vi "Process_EventLogger.vi"(8 "error in (no error)":errorcluster, 10 "MainApplication":refnum<class "MainApplication.lvclass">, 11 "Event Logger in":refnum<class "EventLogger.lvclass">) -> (0 "error out":errorcluster, 3 "Event Logger out":refnum<class "EventLogger.lvclass">)   [LabVIEW 2015, in "EventLogger.lvclass"]
uses:
  EventLogger.lvclass
  MainApplication/MainApplication.lvclass
  MainApplication/MainApplication.lvclass/MainApplication.ctl
  Controls/ChildToAppEventData.ctl
  MainApplication/Accessors/Read AppControlEvents.vi
  MainApplication/Accessors/Read MasterConfig.vi
  MainApplication/Accessors/Read QueueRefnums.vi
  MainApplication/Accessors/Read Dynamic CVT DVR.vi
  DAQ/DAQ.lvclass
  KDC/KDC.lvclass
  Shutter/Shutter.lvclass
  Laser/Laser.lvclass
  LinearStage/LinearStage.lvclass
  PowerMeter/PowerMeter.lvclass
  SystemUI/SystemUI.lvclass
  ChopperWheel/ChopperWheel.lvclass
  KST/KST.lvclass
panel:
  in  "StopLog":bool
  in  "StartLog":bool
  in  "OK":bool
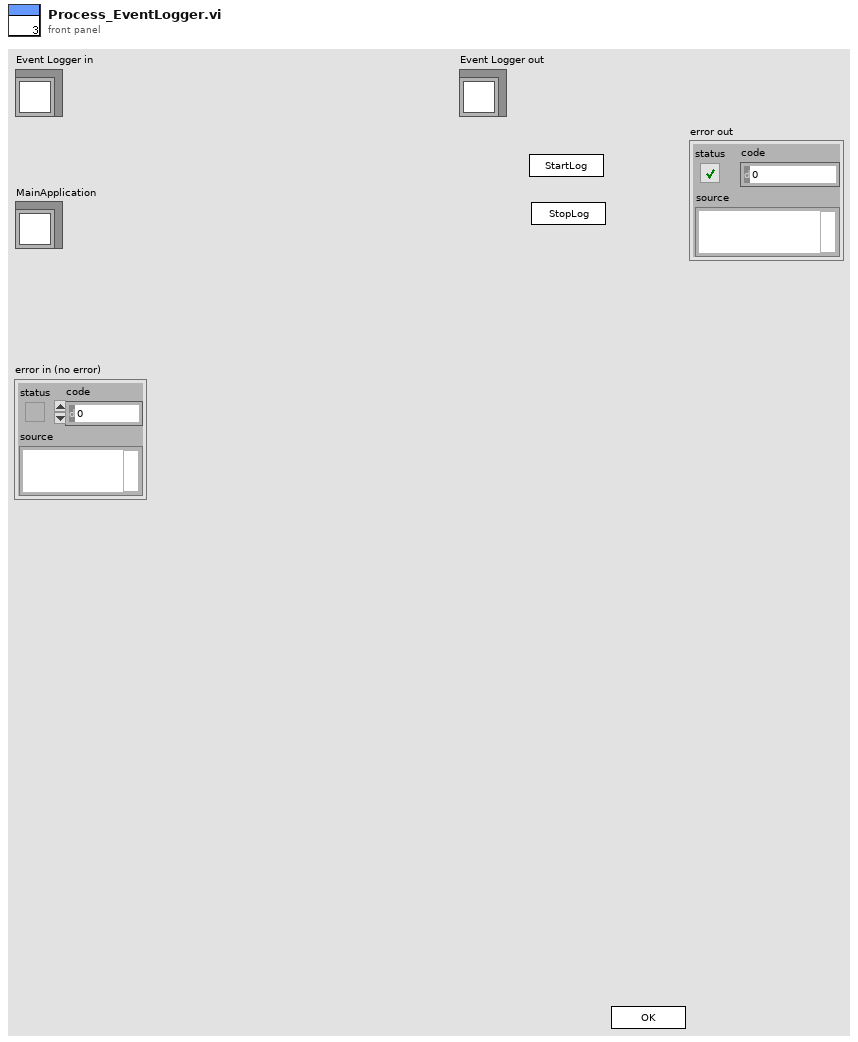
[diagram p1: front panel]
types:
  T1 = typedef "ChildToAppEventData.ctl" = cluster{"Command":string, "Data":variant}
  T2 = enum32{"invalid app kind", "Development System", "Run Time System", "Student Edition", "Embedded LabVIEW", "Evaluation", "Custom"}
  T3 = enum32{"Invalid", "Standard", "Closed", "Hidden", "Minimized", "Maximized"}
  T4 = typedef "PublicEvents--Cluster.ctl" = cluster{"AppToChildEvent":refnum<user-event>, "ChildToAppEvent":refnum<user-event>}
  T5 = typedef "MasterConfiguration--Cluster.ctl" = cluster{"MainAppConfiguration":T6, "ShutterConfiguration":T10, "KDCConfiguration":T12, "DAQConfiguration":T14, "LaserConfiguration":T18, "StageConfiguration":T20, "PowerMeterConfiguration":T22, "SystemUIConfiguration":T24, "ChopperWheelConfiguration":T26, "KSTConfiguration":T28, "Imaging":T30, "EventLoggerConfiguration":T31}
  T6 = typedef "MainAppConfiguration--Cluster.ctl" = cluster{"Simulate":bool, "Station Enable":T7, "StationNames":T8, "CustomScriptConfig":T9[], "C50":bool}
  T7 = typedef "StationEnable--Cluster.ctl" = cluster{"Station 1":bool, "Station 2":bool, "Station 3":bool, "Station 4":bool}
  T8 = typedef "StationModuleNames--Cluster.ctl" = cluster{"Station1Names":string[], "Station2Names":string[], "Station3Names":string[], "Station4Names":string[]}
  T9 = typedef "ScriptButtonConfig--cluster.ctl" = cluster{"OnScriptTitle":string, "OffScriptTitle":string, "OnScriptPath":path, "OffScriptPath":path}
  T10 = typedef "ShutterConfiguration--Cluster.ctl" = cluster{"Shutters":T11[]}
  T11 = typedef "SC10Config--Cluster.ctl" = cluster{"DeviceName":string, "Port":string, "Simulate":bool}
  T12 = typedef "KDC_Configuration--Cluster.ctl" = cluster{"KDC":T13[]}
  T13 = typedef "KDCConfig.ctl" = cluster{"SN":string, "S":dbl, "P":dbl, "Q":dbl, "DeviceName":string, "Simulation":bool, "Offset":dbl}
  T14 = typedef "DAQConfiguration--Cluster.ctl" = cluster{"DAQ":T15[], "Channels":T16[], "DOChannels":T17[]}
  T15 = typedef "DCON_Config--Cluster.ctl" = cluster{"Simulate":bool, "COM":refnum<visa-resource-name>, "baud":u32}
  T16 = typedef "ChannelProperties--Cluster.ctl" = cluster{"Name":string, "DeviceNo":string, "ChannelNo":string, "Active":bool}
  T17 = typedef "DO Channel Info--Cluster.ctl" = cluster{"Name":string, "DeviceNo":string, "GroupNo":string, "Active":bool}
  T18 = typedef "LaserConfiguration--Cluster.ctl" = cluster{"Laser":T19, "LaserLogFolderPath":path, "LaserLogNamePrefix":string, "LaserLogFileInterval_min":dbl, "LaserLogDataInterval_s":dbl}
  T19 = typedef "LaserConfig--Cluster.ctl" = cluster{"DeviceName":string, "Port":string, "Simulate":bool}
  T20 = typedef "LinearStageConfiguration--Cluster.ctl" = cluster{"Stage":T21}
  T21 = typedef "Stage_Config--Cluster.ctl" = cluster{"Simulate":bool, "COM":refnum<visa-resource-name>, "baud":u32}
  T22 = typedef "PowerMeterConfiguration--Cluster.ctl" = cluster{"PowerMeters":T23[], "DataFolderPath":path, "FileNamePrefix":string}
  T23 = typedef "PowerMeterDeviceConfig--Cluster.ctl" = cluster{"DeviceName":string, "SerialNumber":string, "Simulate":bool}
  T24 = typedef "SystemUIConfiguration--Cluster.ctl" = cluster{"Simulate":bool, "SystemUIParameters":T25}
  T25 = typedef "SystemUIParameters--Cluster.ctl" = cluster{"X center":dbl, "Y center":dbl, "X Size":dbl, "Y Size":dbl, "Gap Between Rows":dbl, "Gap Between Columns":dbl, "Gap Between Stage and Stations":dbl, "ConfigType":enum16{"Single-8", "Quad-8", "Quad-16"}}
  T26 = typedef "ChopperWheelConfiguration--Cluster.ctl" = cluster{"ChopperWheel":T27[]}
  T27 = typedef "MC2000B_DevConfig--Cluster.ctl" = cluster{"DeviceName":string, "COMPort":string, "Simulate":bool}
  T28 = typedef "KST_Configuration--Cluster.ctl" = cluster{"KST":T29[]}
  T29 = typedef "KSTConfig.ctl" = cluster{"SN":string, "S":dbl, "P":dbl, "Q":dbl, "DeviceName":string, "Simulation":bool, "Offset":dbl}
  T30 = typedef "Imaging--Cluster.ctl" = cluster{"Cam1":string, "Cam 2":string, "Cam 3":string}
  T31 = typedef "EventLogger_Configuration--Cluster.ctl" = cluster{"LogFolderPath":path}
  T32 = cluster{"Core":cluster{"Current VI Reference":refnum<vi>, "Close Panel on Exit?":bool}, "Event Logger in":refnum<class "EventLogger.lvclass">, "AppControlEvents":T4, "MasterConfiguration*":T5, "LaserConfiguration":T18, "Running":bool}
  T33 = cluster{"Current VI Reference":refnum<vi>, "Close Panel on Exit?":bool}
  T34 = typedef "MS Queue Cluster.ctl" = cluster{"MainQ":refnum<queue>, "StagesQ":refnum<queue>, "ShutterQ":refnum<queue>, "ZaberQ":refnum<queue>, "LaserD":refnum<queue>, "KDCQ":refnum<queue>, "Station 1":refnum<queue>, "Station 2":refnum<queue>, "Station 3":refnum<queue>, "Station 4":refnum<queue>, "PowerMeter":refnum<queue>, "DAQ":refnum<queue>, "CW":refnum<queue>, "KST":refnum<queue>, "EventLogger":refnum<queue>}
  T35 = typedef "TD Dynamic CVT DVR--ref.ctl" = refnum<data-value>
  T36 = cluster{"log file path":path, "Dynamic CVT":T35, "LogFolderPath":path, "Headers in Logfile":string[]}
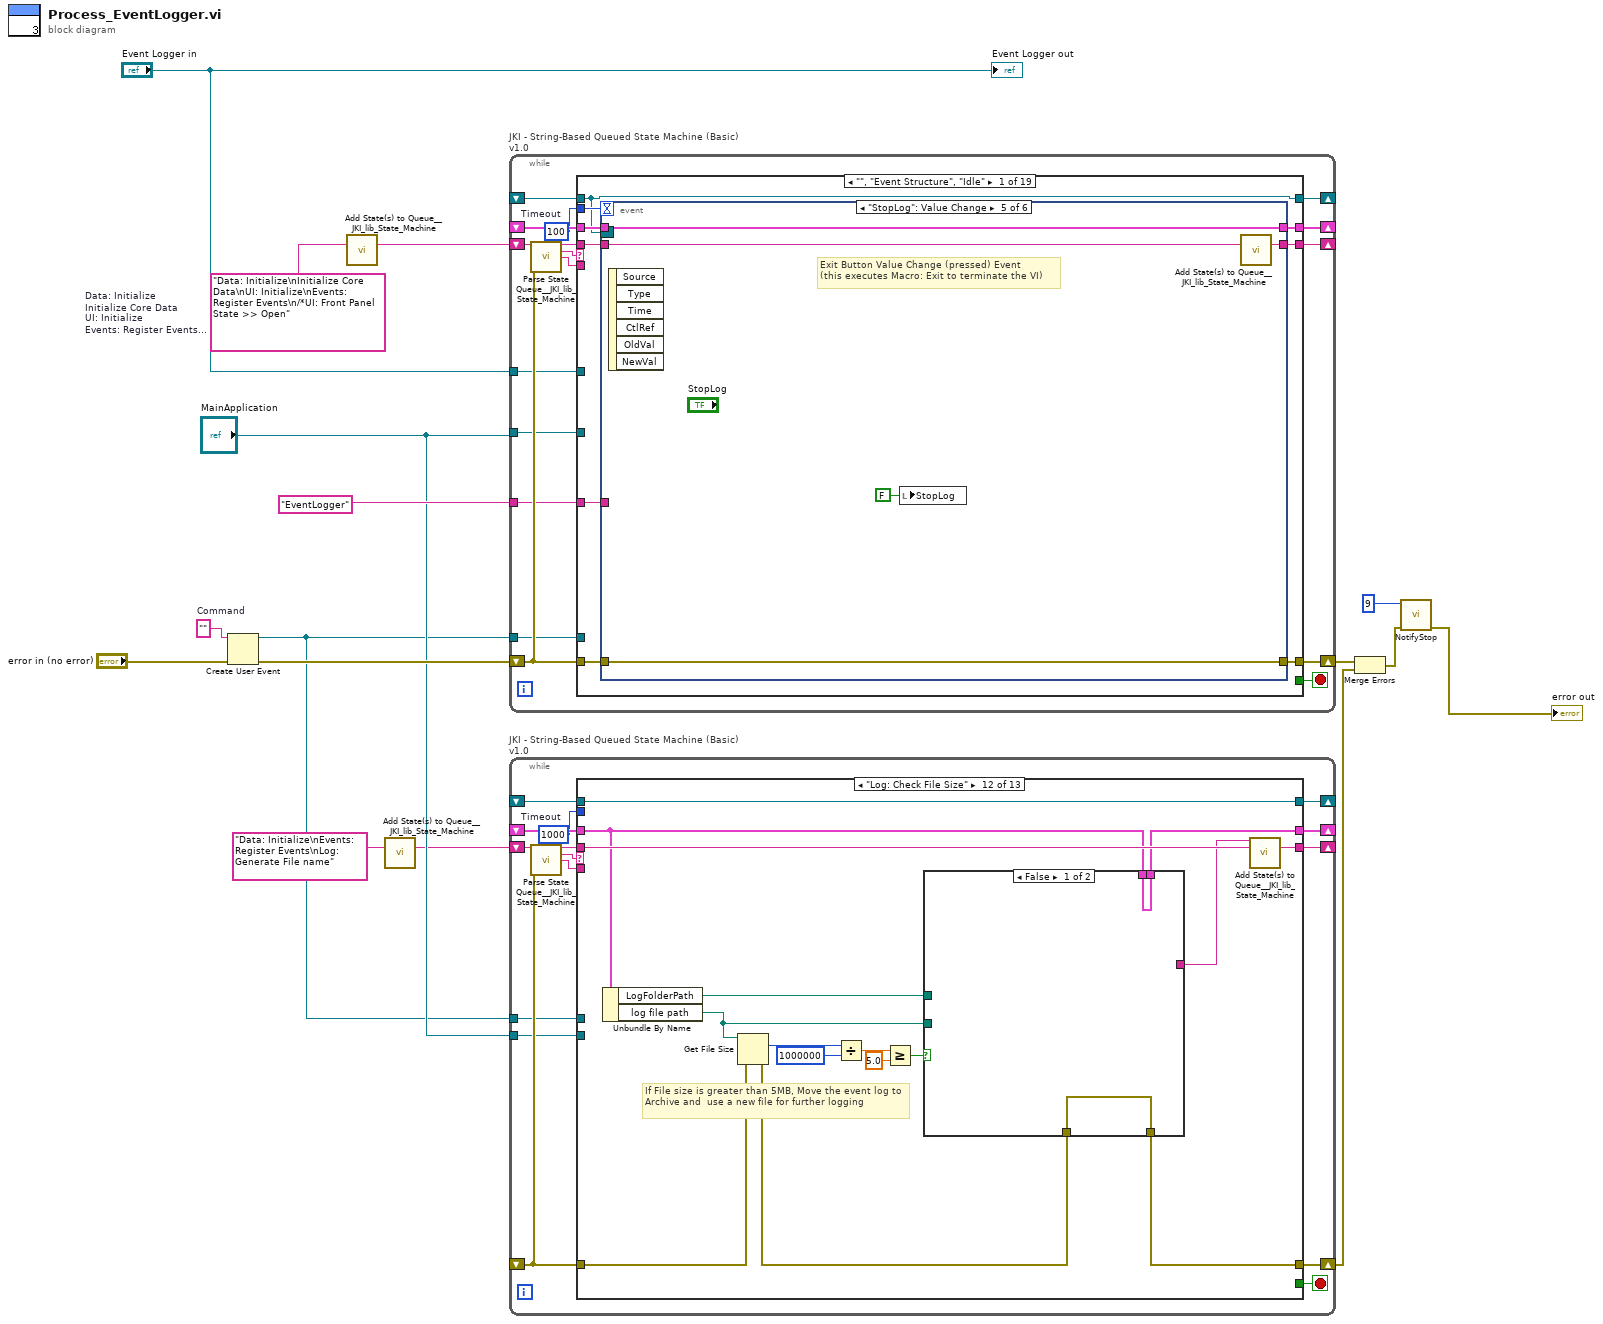
[diagram p0: block diagram]
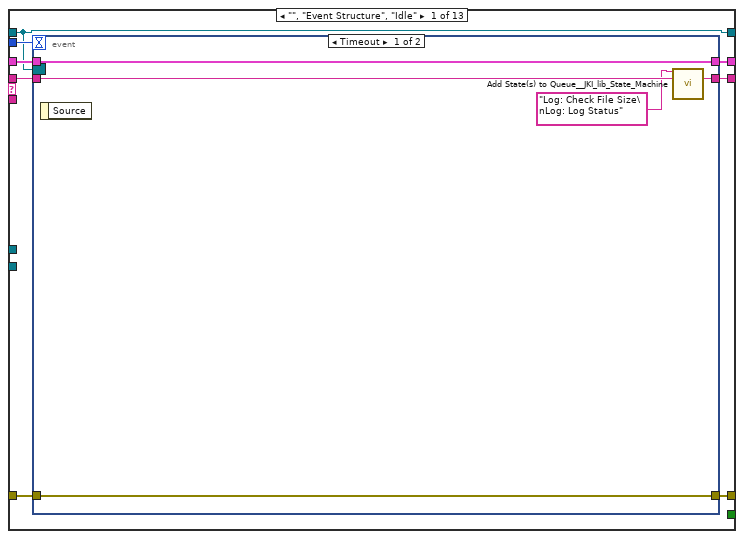
[diagram p2: hidden frame]
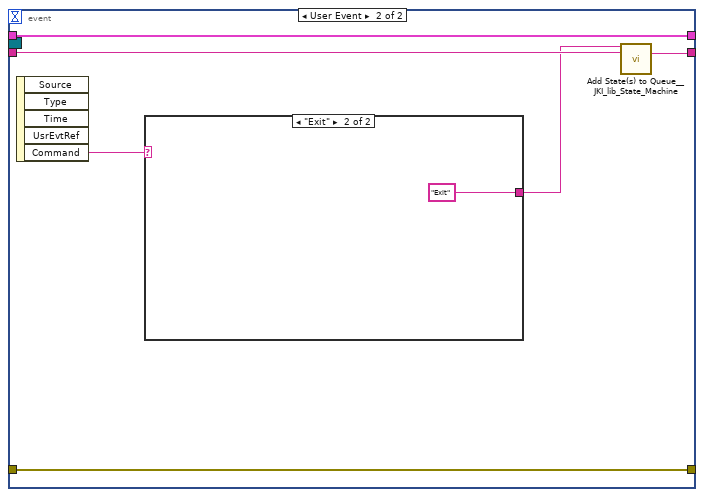
[diagram p3: hidden frame]
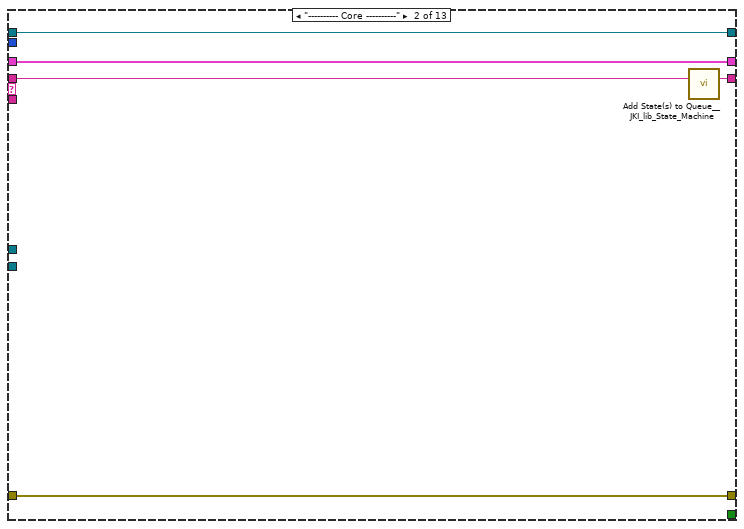
[diagram p5: hidden frame]
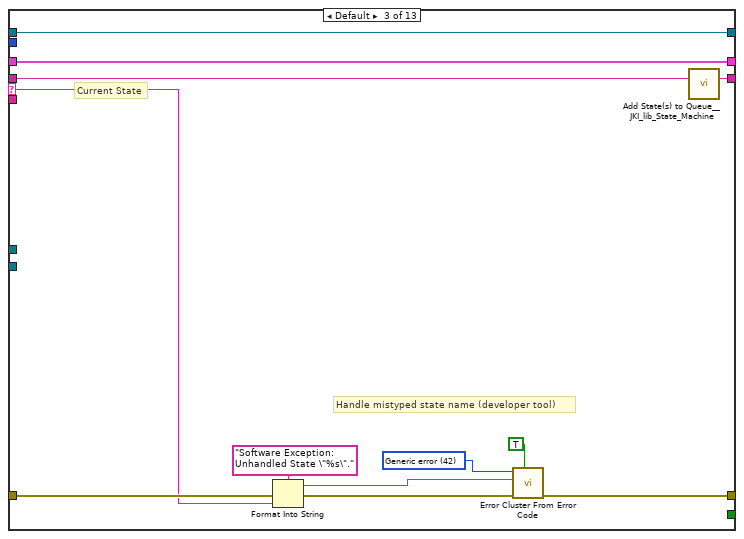
[diagram p6: hidden frame]
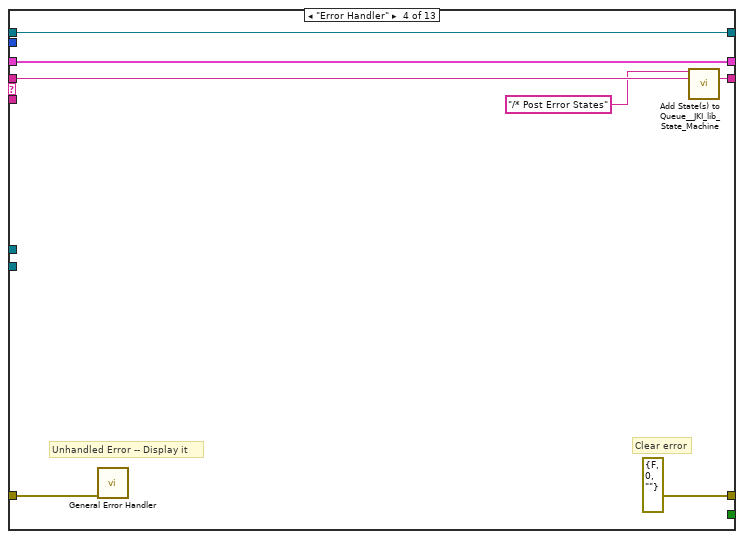
[diagram p7: hidden frame]
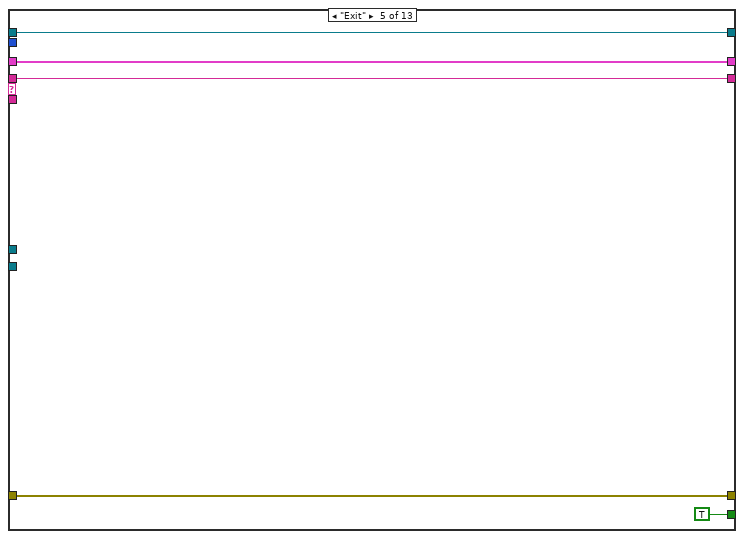
[diagram p8: hidden frame]
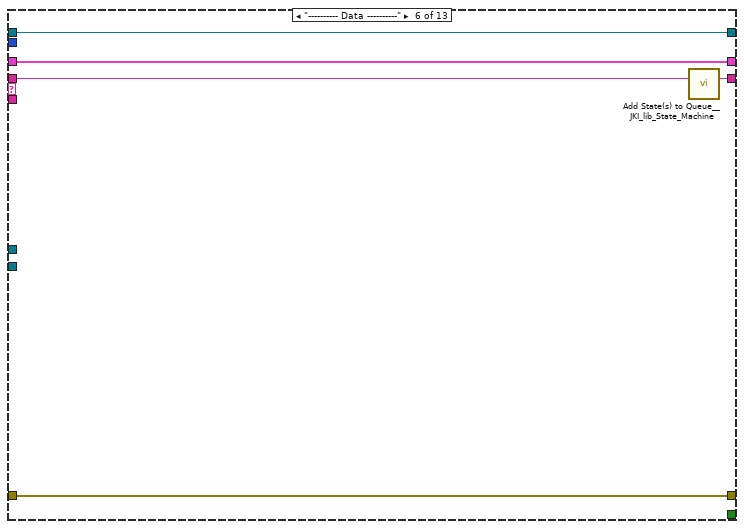
[diagram p9: hidden frame]
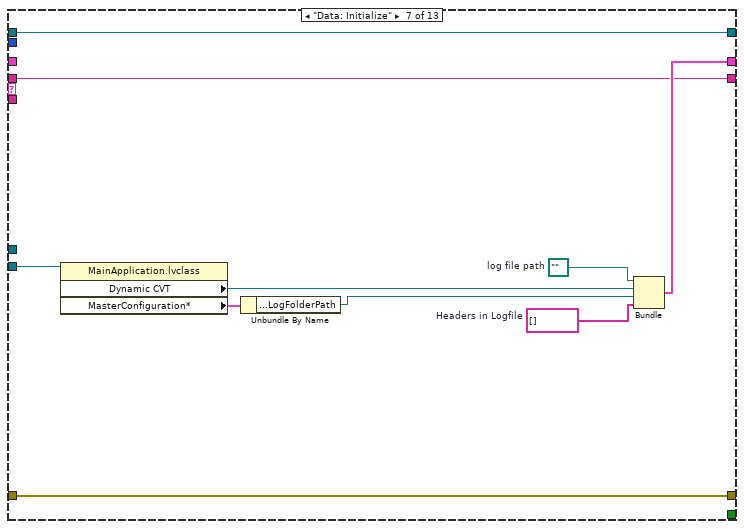
[diagram p10: hidden frame]
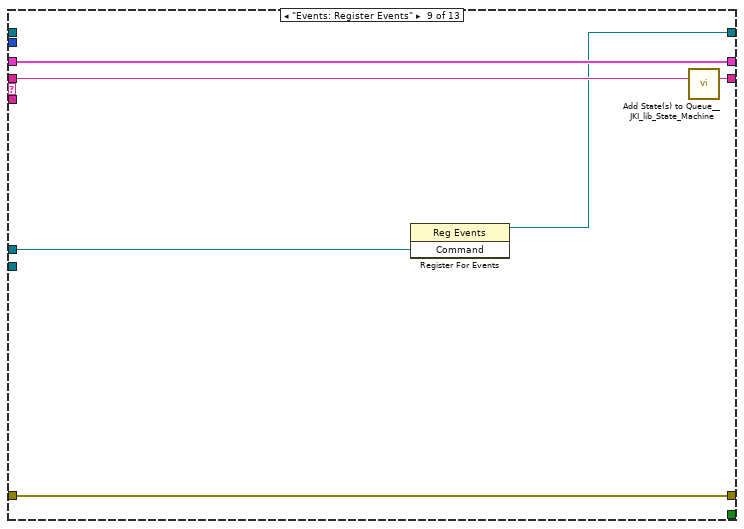
[diagram p12: hidden frame]
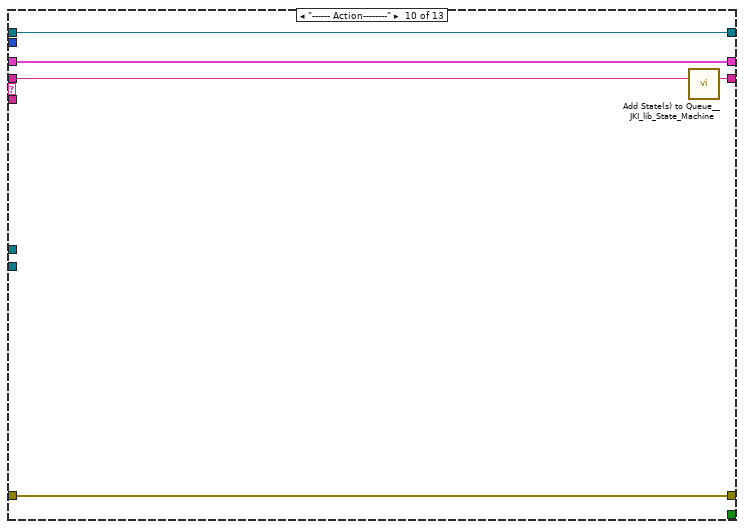
[diagram p13: hidden frame]
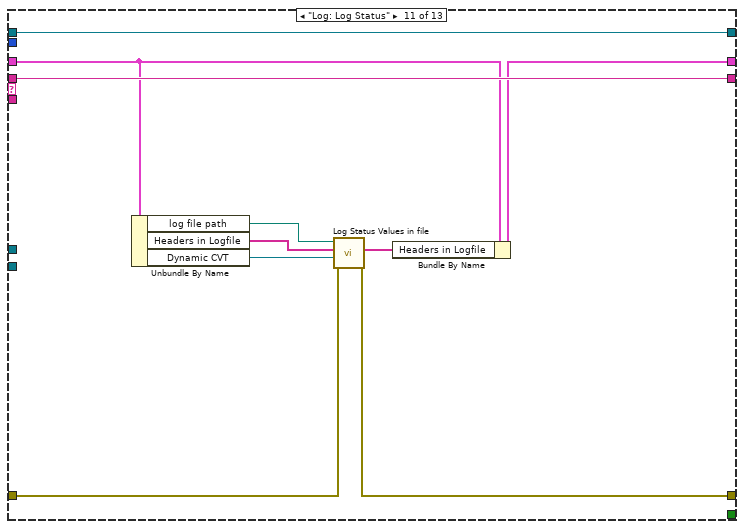
[diagram p14: hidden frame]
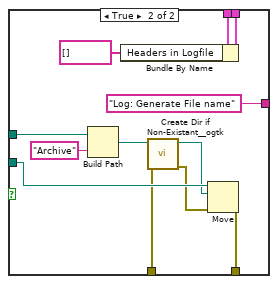
[diagram p15: hidden frame]
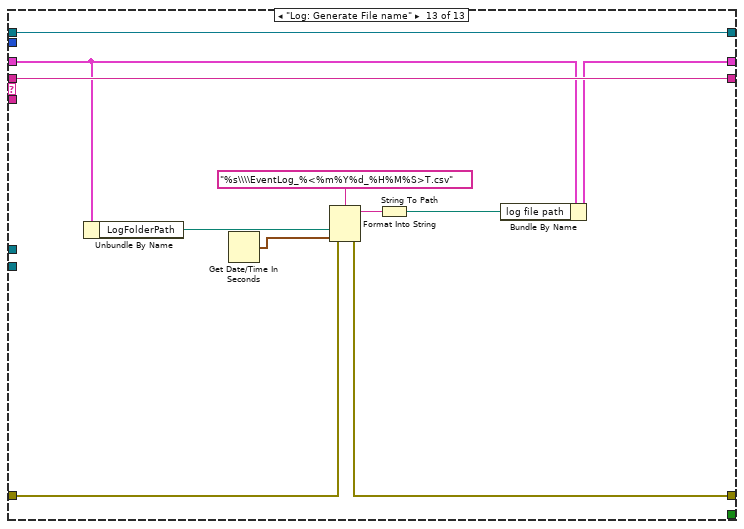
[diagram p16: hidden frame]
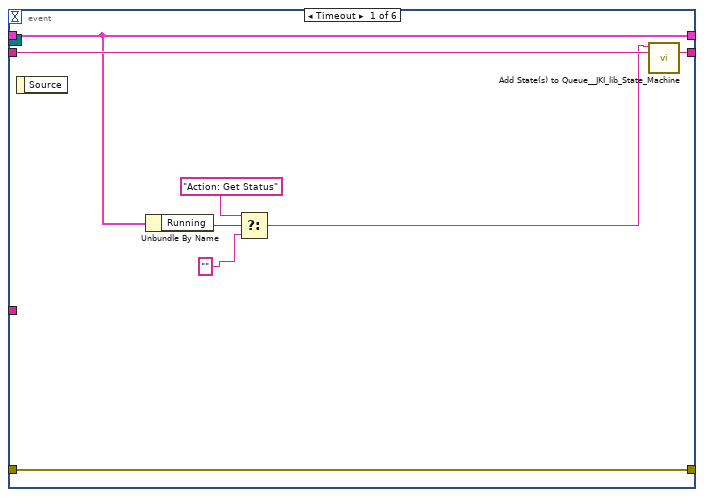
[diagram p17: hidden frame]
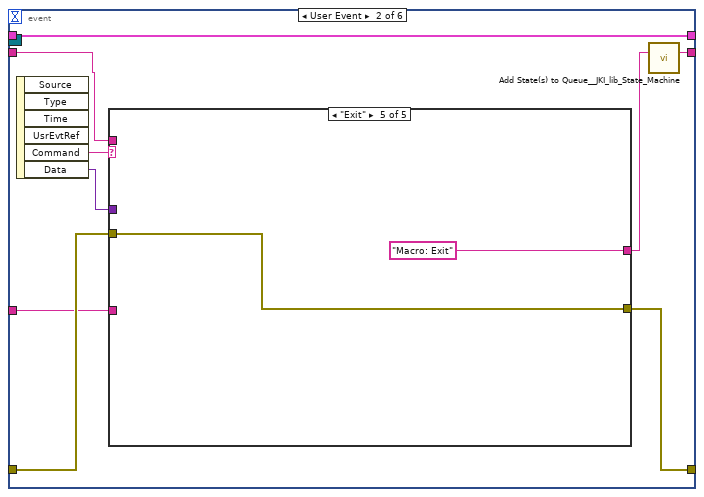
[diagram p18: hidden frame]
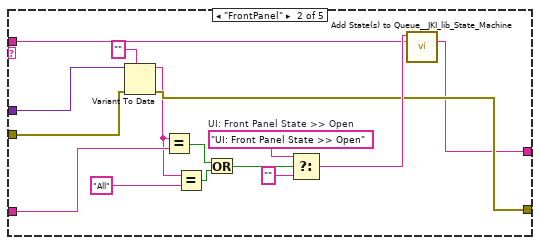
[diagram p20: hidden frame]
diagram:
  w8 = ""  # Command
  w16 = "Data: Initialize\nInitialize Core Data\nUI: Initialize\nEvents: Register Events\n/*UI: Front Panel State >> Open"  # Data: Initialize Initialize Core Data UI: Initialize Events: Register Events /*UI: Front Panel State >> Open
  n1 = Create User Event(user event datatype=w8, error in="error in (no error)") -> (user event=w4:refnum<user-event>, error out=w9:errorcluster)
  n2 = call <vilib>:"Add State(s) to Queue__JKI_lib_State_Machine.vi"("State(s) in (\"\")"=w16) -> ("States Out"=w15:string)  [unwired: 14 in]
  n3 = call <vilib>:"Add State(s) to Queue__JKI_lib_State_Machine.vi"("State(s) in (\"\")"="Data: Initialize\nEvents: Register Events\nLog: Generate File name") -> ("States Out"=w5:string)  [unwired: 14 in]
  n4 = while "JKI - String-Based Queued State Machine (Basic) v1.0" {
    shift-right: [w26] -> _
    shift-left: _ -> [w25]
    shift-right: [w29] -> w3
    shift-left: w9 -> [w23]
    shift-right: [w28] -> _
    shift-left: w15 -> [w30]
    tunnel: "Event Logger in" -> [w22]
    tunnel: "MainApplication" -> [w21]
    shift-right: [w20] -> _
    shift-left: _ -> [w19]
    tunnel: "EventLogger" ("SelfName") -> [w18]
    tunnel: w4 -> [w17]
    stop <- w27 stop-if-true
    w24 = 100  # Timeout
    n5 = call <vilib>:"Parse State Queue__JKI_lib_State_Machine.vi"("State Queue"=w30, "Error In (no error)"=w23) -> ("Remaining States"=w32:string, "Current State"=w33:string, "Arguments"=w31:string)  [unwired: 11 in]
    n6 = case shown="\"\", \"Event Structure\", \"Idle\"" w33 {
      selector: w33 -> [_ _ w120 _ _ _ _ _ _ _ _ _ _ _ _ _ _ _ _]
      tunnel: w32 -> [w42 w118 w124 w143 w150 w156 w161 w175 w185 w190 w196 w203 w215 w244 w255 w259 w265 w270 w281]
      tunnel: w31 -> [_ _ _ _ _ _ _ _ _ _ _ w198 w209 _ _ _ _ _ w272]
      tunnel: w25 -> [w40 w115 w122 w134 w147 w154 w158 _ w181 w187 w194 w201 w211 w241 w252 w257 w261 w267 w278]
      tunnel: [w39 w116 w126 w140 errorcluster {"status"=FALSE, "code"=0, "source"=""} ("error out") w151 w159 w162 w182 w188 w191 w199 w212 w242 w253 w258 w263 w268 w279] -> w29
      tunnel: w23 -> [w38 w116 w125 w140 w146 w151 w159 w162 w178 w188 w192 w200 w213 w242 w253 w258 w263 w268 w279]
      tunnel: [w41 w117 w123 w142 w149 w155 w160 w174 w184 w189 w195 w202 w214 w243 w254 w259 w264 w269 w280] -> w28
      tunnel: [_ _ _ _ _ TRUE _ _ _ _ _ _ _ _ _ _ _ _ _] -> w27
      tunnel: [w37 w115 w122 w141 w147 w154 w158 w173 w181 w187 w194 w201 w211 w241 w252 w257 w261 w267 w278] -> w26
      tunnel: w24 -> [w36 _ _ _ _ _ _ _ _ _ _ _ _ _ _ _ _ _ _]
      tunnel: w22 -> [_ _ _ _ _ _ _ w171 _ _ _ _ _ _ _ _ _ _ _]
      tunnel: w21 -> [_ _ _ _ _ _ _ w170 _ _ _ _ _ w239 _ _ _ _ _]
      tunnel: [w35 w114 w119 w131 w144 w152 w157 w168 w180 w186 w193 w197 w208 w240 w245 w256 w260 w266 w277] -> w20
      tunnel: w19 -> [w35 w114 w119 w131 w144 w152 w157 w168 w180 w186 w193 w197 w208 w240 w245 w256 _ w266 w277]
      tunnel: w18 -> [w34 _ _ _ _ _ _ _ _ _ _ _ _ _ _ _ _ _ _]
      tunnel: w17 -> [_ _ _ _ _ _ _ _ w179 _ _ _ _ _ _ _ _ _ _]
      frame "", "Event Structure", "Idle" {
        n7 = event shown="[4] \"StopLog\": Value Change" {
          selector: w35 -> [_ _ _ _ _ _]
          dyn-events: _ -> [_ _ _ _ _ _]
          timeout: w36 -> [_ _ _ _ _ _]
          tunnel: w42 -> [w50 w53 w99 w104 w109 w113]
          tunnel: [w49 w59 w98 w103 w108 w112] -> w41
          tunnel: w40 -> [w47 w58 w96 w102 w107 w110]
          tunnel: [w48 w54 w97 w101 w106 w111] -> w39
          tunnel: w38 -> [w48 w55 w97 w101 w106 w111]
          tunnel: [w47 w58 w96 w102 w107 w110] -> w37
          tunnel: w34 -> [_ w51 _ _ _ _]
          event Timeout {
            n8 = event-data() -> ()  [unwired: 1 in, 1 out]
            n9 = Unbundle By Name(w47) -> ("Running"=w46:bool)
            n10 = Select(t="Action: Get Status", s=w46, f="") -> (s? t:f=w43:string)
            n11 = call <vilib>:"Add State(s) to Queue__JKI_lib_State_Machine.vi"("State(s) in Front (\"\")"=w43, "State(s) in (\"\")"=w50) -> ("States Out"=w49:string)  [unwired: 13 in]
          }
          event User Event {
            n12 = event-data() -> ("Command"=w57:string, "Data"=w56:variant)  [unwired: 1 in, 4 out]
            n13 = case shown="\"Exit\"" w57 {
              tunnel: [w60 w67 _ w78 "Macro: Exit"] -> w52
              tunnel: w56 -> [_ w72 _ w82 _]
              tunnel: w55 -> [w61 w71 w77 w81 w93]
              tunnel: [w61 w70 w77 w80 w93] -> w54
              tunnel: w53 -> [w60 w68 _ w79 _]
              tunnel: w51 -> [_ w69 _ _ _]
              frame "False", Default {
              }
              frame "FrontPanel" {
                w75 = "UI: Front Panel State >> Open"  # UI: Front Panel State >> Open
                n14 = Variant To Data(error in=w71, type="", Variant=w72) -> (data=w64:string, error out=w70:errorcluster)
                n15 = Equal?(x=w64, y=w69) -> (x = y?=w63:bool)
                n16 = Equal?(x=w64, y="All") -> (x = y?=w65:bool)
                n17 = Or(x=w63, y=w65) -> (x .or. y?=w62:bool)
                n18 = Select(t=w75, s=w62, f="") -> (s? t:f=w73:string)
                n19 = call <vilib>:"Add State(s) to Queue__JKI_lib_State_Machine.vi"("State(s) in Front (\"\")"=w73, "State(s) in (\"\")"=w68) -> ("States Out"=w67:string)  [unwired: 13 in]
              }
              frame "Abort" {
              }
              frame "EventLogger" {
                n20 = Variant To Data(error in=w81, type=T1 {"Command"="", "Data"=variant} ("event data"), Variant=w82) -> (data=w86:T1, error out=w87:errorcluster)
                n21 = Unbundle By Name(w86) -> ("Data"=w85:variant, "Command"=w89:string)
                n22 = Variant To Data(error in=w87, type="", Variant=w85) -> (data=w88:string, error out=w92:errorcluster)
                n23 = Format Into String(format string="Execute Command>>%s>>%s", error in=w92, w88, w89) -> (resulting string=w90:string, error out=w80:errorcluster)  [unwired: 1 in]
                n24 = call <vilib>:"Add State(s) to Queue__JKI_lib_State_Machine.vi"("State(s) in (\"\")"=w79, "State(s) at Back (\"\")"=w90) -> ("States Out"=w78:string)  [unwired: 13 in]
              }
              frame "Exit" {
              }
            }
            n25 = call <vilib>:"Add State(s) to Queue__JKI_lib_State_Machine.vi"("State(s) in (\"\")"=w52) -> ("States Out"=w59:string)  [unwired: 14 in]
          }
          event "OK": Value Change {
            # "Exit Button Value Change (pressed) Event\n(this executes Macro: Exit to terminate the VI)"
            n26 = event-data() -> ()  [unwired: 1 in, 1 out]
            n27 = call <vilib>:"Add State(s) to Queue__JKI_lib_State_Machine.vi"("State(s) in Front (\"\")"="Macro: Exit", "State(s) in (\"\")"=w99) -> ("States Out"=w98:string)  [unwired: 13 in]
          }
          event "StartLog": Value Change {
            # "Exit Button Value Change (pressed) Event\n(this executes Macro: Exit to terminate the VI)"
            n28 = event-data() -> ()  [unwired: 1 in, 6 out]
            n29 = local write "StartLog"(FALSE ("StartLog")) -> ()
            n30 = call <vilib>:"Add State(s) to Queue__JKI_lib_State_Machine.vi"("State(s) in (\"\")"=w104) -> ("States Out"=w103:string)  [unwired: 14 in]
          }
          event "StopLog": Value Change {
            # "Exit Button Value Change (pressed) Event\n(this executes Macro: Exit to terminate the VI)"
            n31 = event-data() -> ()  [unwired: 1 in, 6 out]
            n32 = local write "StopLog"(FALSE ("StopLog")) -> ()
            n33 = call <vilib>:"Add State(s) to Queue__JKI_lib_State_Machine.vi"("State(s) in (\"\")"=w109) -> ("States Out"=w108:string)  [unwired: 14 in]
          }
          event Panel Close? {
            # "Close Panel button (pressed) Event\n(this executes Macro: Exit to terminate the VI)"
            n34 = event-data() -> ()  [unwired: 1 in, 1 out]
            n35 = event-data() -> ()  [unwired: 2 in, 1 out]
            n36 = call <vilib>:"Add State(s) to Queue__JKI_lib_State_Machine.vi"("State(s) in (\"\")"=w113) -> ("States Out"=w112:string)  [unwired: 14 in]
          }
        }
      }
      frame "---------- Core ----------" {
        n37 = call <vilib>:"Add State(s) to Queue__JKI_lib_State_Machine.vi"("State(s) in (\"\")"=w118) -> ("States Out"=w117:string)  [unwired: 14 in]
      }
      frame Default {
        w129 = 42 items=["No error", "Argument error", "Memory is full", "Out of zone", "End of file", "File already open", "Generic file I/O error", "File not found", "File permission error", "Disk is full", "Duplicate path", "Too many files open", "System feature not enabled", "Resource file not found", "Cannot add resource", "Resource not found", "Image not found", "Image memory error", "Pen does not exist", "Config type invalid", "Config token not found", "Config parse error", "Config memory error", "Bad external code format", "Bad external code offset", "External code not present", "Null window", "Destroy window error", "Null menu", "Print aborted", "Bad print record", "Print driver error", "Windows error during printing", "Memory error during printing", "Print dialog error", "Generic print error", "Invalid device refnum", "Device not found", "Device parameter error", "Device unit error", "Cannot open device", "Device call aborted", "Generic error", "Cancelled by user", "Object ID too low", "Object ID too high", "Object not in heap", "Unknown heap", "Unknown object (invalid DefProc)", "Unknown object (DefProc not in table)", "Message out of range", "Invalid (null) method", "Unknown message", "Manager call not supported", "Bad address", "Network operation in progress", "Network operation timed out", "Connection is busy", "Network attribute not supported", "Network error", "Address in use", "System out of memory", "Connection aborted", "Connection refused", "Not connected", "Already connected", "Connection closed", "Initialization error (interapplication manager)", "Bad occurrence", "Wait on unbound occurrence handler", "Occurrence queue overflow", "Datalog type conflict", "Unused", "Unrecognized type (interapplication manager)", "Memory corrupt", "Failed to make temporary DLL", "Old CIN version", "Drag socket not found", "Failed to load drop-object", "Failed to register OLE object", "Failed to release OLE object", "Format specifier type mismatch", "Unknown format specifier", "Too few format specifiers", "Too many format specifiers", "Scan failed", "Newer CIN version", "Error converting to variant", "Runtime menu error", "Password tampered", "Variant attribute not found", "Incompatible variant data type", "Event data is not available", "Event Store is not present", "Occurrence is not found", "Event Queue is not created", "Event info is not available", "Refnum passed is NULL", "Error retrieving Class GUID", "Error retrieving CoClass GUID", "Error retrieving TypeLib GUID.", "Bad built application magic bytes.", "Specific driver is different from the specific driver associated with the Logical Name.", "There is no session opened to the class driver.", "Max Error", "MAX - Error with config objects", "MAX - Error loading configuration", "MAX - Group not supported"]
        # "Current State"
        # "Handle mistyped state name (developer tool)"
        n38 = Format Into String(format string="Software Exception: Unhandled State \"%s\"." ("message"), error in=w125, w120) -> (resulting string=w128:string, error out=w127:errorcluster)  [unwired: 1 in]
        n39 = call <vilib>:"Error Cluster From Error Code.vi"("show call chain? (False)"=TRUE, "error in (no error)"=w127, "error message (\"\")"=w128, "error code (0)"=w129) -> ("error out"=w126:errorcluster)  [unwired: 5 in]
        n40 = call <vilib>:"Add State(s) to Queue__JKI_lib_State_Machine.vi"("State(s) in (\"\")"=w124) -> ("States Out"=w123:string)  [unwired: 14 in]
      }
      frame "Initialize Core Data" {
        # "originally closed?"
        # "exe?"
        # "If panel starts closed or is an EXE, then close it when we exit"
        n41 = property class="VI"() -> ("Front Panel.Open"=w139:bool)  [unwired: 2 in, 2 out]
        n42 = property class="App"() -> ("App.Kind"=w138:T2)  [unwired: 2 in, 2 out]
        n43 = control-ref of="Current VI Reference"() -> (w132:refnum<vi>)
        n44 = Not(x=w139) -> (.not. x?=w136:bool)
        n45 = Equal?(x=w138, y=T2."Run Time System" ("Application:Kind")) -> (x = y?=w135:bool)
        n46 = Or(x=w136, y=w135) -> (x .or. y?=w133:bool)
        n47 = Bundle By Name(cluster=w134, "Core.Current VI Reference"=w132, "Core.Close Panel on Exit?"=w133) -> (w141:T32)
        n48 = call <vilib>:"Add State(s) to Queue__JKI_lib_State_Machine.vi"("State(s) in (\"\")"=w143) -> ("States Out"=w142:string)  [unwired: 14 in]
      }
      frame "Error Handler" {
        # "Unhandled Error -- Display it"
        # "Clear error"
        n49 = call <vilib>:"General Error Handler.vi"("error in (no error)"=w146) -> ()  [unwired: 10 in, 5 out]
        n50 = call <vilib>:"Add State(s) to Queue__JKI_lib_State_Machine.vi"("State(s) in Front (\"\")"="/* Post Error States", "State(s) in (\"\")"=w150) -> ("States Out"=w149:string)  [unwired: 13 in]
      }
      frame "Exit" {
        n51 = call <vilib>:"Add State(s) to Queue__JKI_lib_State_Machine.vi"("State(s) in (\"\")"=w156) -> ("States Out"=w155:string)  [unwired: 14 in]
      }
      frame "---------- Data ----------" {
        n52 = call <vilib>:"Add State(s) to Queue__JKI_lib_State_Machine.vi"("State(s) in (\"\")"=w161) -> ("States Out"=w160:string)  [unwired: 14 in]
      }
      frame "Data: Initialize" {
        w165 = FALSE  # Running
        w172 = T33 {"Current VI Reference"=refnum, "Close Panel on Exit?"=FALSE}  # Core
        n53 = property class="MainApplication.lvclass"(reference=w170) -> ("AppControlEvents"=w169:T4, "MasterConfiguration*"=w166:T5, "MasterConfiguration*"=w167:T5, "QueueRefnums*"=w163:T34)  [unwired: 1 in, 2 out]
        n54 = Unbundle By Name(w167) -> ("LaserConfiguration"=w164:T18)
        n55 = Unbundle By Name(w163) -> ()  [unwired: 1 out]
        n56 = Bundle("Core"=w172, "Event Logger in"=w171, "AppControlEvents"=w169, "MasterConfiguration*"=w166, "LaserConfiguration"=w164, "Running"=w165) -> (w173:T32)  [unwired: 1 in]
        n57 = call <vilib>:"Add State(s) to Queue__JKI_lib_State_Machine.vi"("State(s) in (\"\")"=w175) -> ("States Out"=w174:string)  [unwired: 14 in]
      }
      frame "Data: Cleanup" {
        n58 = Unbundle By Name(w181) -> ("Core.Current VI Reference"=w183:refnum<vi>)
        n59 = Generate User Event(user event=w179, event data cluster="Exit" ("event data"), error in=w178) -> (error out=w177:errorcluster)  [unwired: 1 in, 1 out]
        n60 = Close Reference(reference=w183, error in (no error)=w177) -> (error out=w182:errorcluster)
        n61 = call <vilib>:"Add State(s) to Queue__JKI_lib_State_Machine.vi"("State(s) in (\"\")"=w185) -> ("States Out"=w184:string)  [unwired: 14 in]
      }
      frame "---------- UI ----------" {
        n62 = call <vilib>:"Add State(s) to Queue__JKI_lib_State_Machine.vi"("State(s) in (\"\")"=w190) -> ("States Out"=w189:string)  [unwired: 14 in]
      }
      frame "UI: Initialize" {
        n63 = call <userlib>:"Fit VI window to Largest Dec__ogtk.vi"("error in (no error)"=w192) -> ("error out"=w191:errorcluster)  [unwired: 5 in, 1 out]
        n64 = call <vilib>:"Add State(s) to Queue__JKI_lib_State_Machine.vi"("State(s) in (\"\")"=w196) -> ("States Out"=w195:string)  [unwired: 14 in]
      }
      frame "UI: Cursor Set" {
        # "Argument"
        n65 = case shown="\"Idle\", Default" w198 {
          tunnel: w200 -> [w205 w207]
          tunnel: [w204 w206] -> w199
          frame "Idle", Default {
            n66 = call <vilib>:"Unset Busy.vi"("error in (no error)"=w205) -> ("error out"=w204:errorcluster)  [unwired: 10 in]
          }
          frame "Busy" {
            n67 = call <vilib>:"Set Busy.vi"("error in (no error)"=w207) -> ("error out"=w206:errorcluster)  [unwired: 9 in, 1 out]
          }
        }
        n68 = call <vilib>:"Add State(s) to Queue__JKI_lib_State_Machine.vi"("State(s) in (\"\")"=w203) -> ("States Out"=w202:string)  [unwired: 14 in]
      }
      frame "UI: Front Panel State" {
        # "Argument"
        n69 = Unbundle By Name(w211) -> ("Core.Current VI Reference"=w210:refnum<vi>)
        n70 = case shown="\"Open\", Default" w209 {
          tunnel: w213 -> [w219 w232]
          tunnel: [w221 w233] -> w212
          tunnel: w210 -> [w220 w230]
          frame "Open", Default {
            n71 = property class="VI"(reference=w220, error in=w219) -> (reference out=w217:refnum<vi>, error out=w218:errorcluster, "Front Panel.Open"=w216:bool)
            n72 = case shown="False" w216 {
              tunnel: [w224 w227] -> w221
              tunnel: w218 -> [w223 w227]
              tunnel: w217 -> [w222 _]
              frame False {
                n73 = invoke class="VI" method="FP.Open"(reference=w222, error in=w223, "Activate"=TRUE, "State"=T3."Standard") -> (error out=w224:errorcluster)  [unwired: 1 in, 4 out]
              }
              frame True {
              }
            }
          }
          frame "Close" {
            n74 = property class="VI"(reference=w230, error in=w232) -> (reference out=w229:refnum<vi>, error out=w231:errorcluster, "Front Panel.Open"=w228:bool)
            n75 = case shown="True" w228 {
              tunnel: [w234 w237] -> w233
              tunnel: w231 -> [w234 w236]
              tunnel: w229 -> [_ w235]
              frame False {
              }
              frame True {
                n76 = invoke class="VI" method="FP.Close"(reference=w235, error in=w236) -> (error out=w237:errorcluster)  [unwired: 1 in, 2 out]
              }
            }
          }
        }
        n77 = call <vilib>:"Add State(s) to Queue__JKI_lib_State_Machine.vi"("State(s) in (\"\")"=w215) -> ("States Out"=w214:string)  [unwired: 14 in]
      }
      frame "---------- Macro ----------" {
        n78 = property class="MainApplication.lvclass"(reference=w239) -> ("QueueRefnums*"=w238:T34)  [unwired: 1 in, 2 out]
        n79 = Unbundle By Name(w238) -> ()  [unwired: 1 out]
        n80 = call <vilib>:"Add State(s) to Queue__JKI_lib_State_Machine.vi"("State(s) in (\"\")"=w244) -> ("States Out"=w243:string)  [unwired: 14 in]
      }
      frame "Macro: Exit" {
        n81 = Unbundle By Name(w252) -> ("Core.Close Panel on Exit?"=w251:bool)
        n82 = Select(t="UI: Front Panel State >> Close", s=w251, f="") -> (s? t:f=w248:string)
        n83 = call <vilib>:"Add State(s) to Queue__JKI_lib_State_Machine.vi"("State(s) in (\"\")"=w248, "State(s) at Back (\"\")"="Data: Cleanup\nExit") -> ("States Out"=w246:string)  [unwired: 13 in]
        n84 = call <vilib>:"Add State(s) to Queue__JKI_lib_State_Machine.vi"("State(s) in Front (\"\")"=w246, "State(s) in (\"\")"=w255) -> ("States Out"=w254:string)  [unwired: 13 in]
      }
      frame "---------- Events ----------" {
      }
      frame "Events: Register Events" {
        n85 = Unbundle By Name(w261) -> ("AppControlEvents.AppToChildEvent"=w262:refnum<user-event>)
        n86 = register-events(w262) -> (reference out=w260:refnum<event-registration>)  [unwired: 2 in, 1 out]
        n87 = call <vilib>:"Add State(s) to Queue__JKI_lib_State_Machine.vi"("State(s) in (\"\")"=w265) -> ("States Out"=w264:string)  [unwired: 14 in]
      }
      frame "------ Action--------" {
        n88 = call <vilib>:"Add State(s) to Queue__JKI_lib_State_Machine.vi"("State(s) in (\"\")"=w270) -> ("States Out"=w269:string)  [unwired: 14 in]
      }
      frame "Execute Command" {
        (unwired) "Action: Wait for Stage Move>>Initialize;%s" ("format string")
        n89 = call <vilib>:"Parse State Queue__JKI_lib_State_Machine.vi"("State Queue"=w272) -> ("Current State"=w274:string, "Arguments"=w273:string)  [unwired: 12 in, 1 out]
        n90 = call <vilib>:"Parse State Queue__JKI_lib_State_Machine.vi"("State Queue"=w273) -> ("Current State"=w275:string, "Arguments"=w276:string)  [unwired: 12 in, 1 out]
        n91 = case shown="\"SetLaserMode\"" w275 {
          tunnel: [_ w282 w292 w302] -> w271
          tunnel: w276 -> [_ w286 w296 w306]
          tunnel: w274 -> [_ w285 w295 w305]
          frame "False", Default {
          }
          frame "SetLaserPower" {
            # "Action: SetLaserOutput>>Script;20"
            # "Stage Move>>Segment;Station 1"
            n92 = Scan From String(format string="%[^;];%s", input string=w286) -> (output 1=w284:string, output 2=w283:string)  [unwired: 4 in, 3 out]
            n93 = case shown="\"Sync\", Default" w285 {
              tunnel: w284 -> [w290 _]
              tunnel: w283 -> [w289 _]
              tunnel: [w288 _] -> w282
              frame "Async" {
                n94 = Format Into String(format string="Action: Set Laser Power>>%s;%s", w290, w289) -> (resulting string=w288:string)  [unwired: 2 in, 1 out]
              }
              frame "Sync", Default {
              }
            }
          }
          frame "SetLaserMode" {
            n95 = Scan From String(format string="%[^;];%s", input string=w296) -> (output 1=w294:string, output 2=w293:string)  [unwired: 4 in, 3 out]
            n96 = case shown="\"Async\"" w295 {
              tunnel: w294 -> [w300 _]
              tunnel: w293 -> [w299 _]
              tunnel: [w298 _] -> w292
              frame "Async" {
                n97 = Format Into String(format string="Action: Set Laser Mode>>%s;%s", w300, w299) -> (resulting string=w298:string)  [unwired: 2 in, 1 out]
              }
              frame "Sync", Default {
              }
            }
          }
          frame "SetLaserShutter" {
            n98 = Scan From String(format string="%[^;];%s", input string=w306) -> (output 1=w304:string, output 2=w303:string)  [unwired: 4 in, 3 out]
            n99 = case shown="\"Async\"" w305 {
              tunnel: w304 -> [w310 _]
              tunnel: w303 -> [w309 _]
              tunnel: [w308 _] -> w302
              frame "Async" {
                n100 = Format Into String(format string="Action: Set Laser Shutter>>%s;%s", w310, w309) -> (resulting string=w308:string)  [unwired: 2 in, 1 out]
              }
              frame "Sync", Default {
              }
            }
          }
        }
        n101 = call <vilib>:"Add State(s) to Queue__JKI_lib_State_Machine.vi"("State(s) in Front (\"\")"=w271, "State(s) in (\"\")"=w281) -> ("States Out"=w280:string)  [unwired: 13 in]
      }
    }
  }
  n102 = while "JKI - String-Based Queued State Machine (Basic) v1.0" {
    shift-right: [w319] -> _
    shift-left: _ -> [w318]
    shift-right: [w322] -> w2
    shift-left: _ -> [w316]
    shift-right: [w321] -> _
    shift-left: w5 -> [w323]
    tunnel: "MainApplication" -> [w315]
    shift-right: [w314] -> _
    shift-left: _ -> [w313]
    tunnel: w4 -> [w312]
    stop <- w320 stop-if-true
    w317 = 1000  # Timeout
    n103 = call <vilib>:"Parse State Queue__JKI_lib_State_Machine.vi"("State Queue"=w323, "Error In (no error)"=w316) -> ("Remaining States"=w325:string, "Current State"=w326:string, "Arguments"=w324:string)  [unwired: 11 in]
    n104 = case shown="\"Log: Check File Size\"" w326 {
      selector: w326 -> [_ _ w353 _ _ _ _ _ _ _ _ _ _]
      tunnel: w325 -> [w334 w351 w357 w370 w375 w380 w381 w394 w400 w405 w410 w420 w450]
      tunnel: w324 -> [_ _ _ _ _ _ _ _ _ _ _ _ _]
      tunnel: w318 -> [w332 w348 w355 w367 w374 w377 _ w392 w397 w402 w407 w417 w447]
      tunnel: [w331 w349 w359 errorcluster {"status"=FALSE, "code"=0, "source"=""} ("error out") w371 w378 w383 w393 w398 w403 w411 w421 w451] -> w322
      tunnel: w316 -> [w330 w349 w358 w366 w371 w378 w383 w393 w398 w403 w412 w430 w452]
      tunnel: [w333 w350 w356 w369 w375 w379 w381 w394 w399 w404 w410 w419 w450] -> w321
      tunnel: [_ _ _ _ TRUE _ _ _ _ _ _ _ _] -> w320
      tunnel: [w329 w348 w355 w367 w374 w377 w385 w392 w397 w402 w406 w416 w446] -> w319
      tunnel: w317 -> [w328 _ _ _ _ _ _ _ _ _ _ _ _]
      tunnel: w315 -> [_ _ _ _ _ _ w390 _ _ _ _ _ _]
      tunnel: [w327 w347 w352 w364 w372 w376 w388 w391 w396 w401 w415 w431 w456] -> w314
      tunnel: w313 -> [w327 w347 w352 w364 w372 w376 w388 w391 _ w401 w415 w431 w456]
      tunnel: w312 -> [_ _ _ _ _ _ _ _ w395 _ _ _ _]
      frame "", "Event Structure", "Idle" {
        n105 = event shown="[0] Timeout" {
          selector: w327 -> [_ _]
          dyn-events: _ -> [_ _]
          timeout: w328 -> [_ _]
          tunnel: w334 -> [w339 w343]
          tunnel: [w338 w342] -> w333
          tunnel: w332 -> [w336 w344]
          tunnel: [w337 w341] -> w331
          tunnel: w330 -> [w337 w341]
          tunnel: [w336 w344] -> w329
          event Timeout {
            n106 = event-data() -> ()  [unwired: 1 in, 1 out]
            n107 = call <vilib>:"Add State(s) to Queue__JKI_lib_State_Machine.vi"("State(s) in Front (\"\")"="Log: Check File Size\nLog: Log Status", "State(s) in (\"\")"=w339) -> ("States Out"=w338:string)  [unwired: 13 in]
          }
          event User Event {
            n108 = event-data() -> ("Command"=w345:string)  [unwired: 1 in, 4 out]
            n109 = case shown="\"Exit\"" w345 {
              tunnel: [_ "Exit"] -> w340
              frame "False", Default {
              }
              frame "Exit" {
              }
            }
            n110 = call <vilib>:"Add State(s) to Queue__JKI_lib_State_Machine.vi"("State(s) in Front (\"\")"=w340, "State(s) in (\"\")"=w343) -> ("States Out"=w342:string)  [unwired: 13 in]
          }
        }
      }
      frame "---------- Core ----------" {
        n111 = call <vilib>:"Add State(s) to Queue__JKI_lib_State_Machine.vi"("State(s) in (\"\")"=w351) -> ("States Out"=w350:string)  [unwired: 14 in]
      }
      frame Default {
        w362 = 42 items=["No error", "Argument error", "Memory is full", "Out of zone", "End of file", "File already open", "Generic file I/O error", "File not found", "File permission error", "Disk is full", "Duplicate path", "Too many files open", "System feature not enabled", "Resource file not found", "Cannot add resource", "Resource not found", "Image not found", "Image memory error", "Pen does not exist", "Config type invalid", "Config token not found", "Config parse error", "Config memory error", "Bad external code format", "Bad external code offset", "External code not present", "Null window", "Destroy window error", "Null menu", "Print aborted", "Bad print record", "Print driver error", "Windows error during printing", "Memory error during printing", "Print dialog error", "Generic print error", "Invalid device refnum", "Device not found", "Device parameter error", "Device unit error", "Cannot open device", "Device call aborted", "Generic error", "Cancelled by user", "Object ID too low", "Object ID too high", "Object not in heap", "Unknown heap", "Unknown object (invalid DefProc)", "Unknown object (DefProc not in table)", "Message out of range", "Invalid (null) method", "Unknown message", "Manager call not supported", "Bad address", "Network operation in progress", "Network operation timed out", "Connection is busy", "Network attribute not supported", "Network error", "Address in use", "System out of memory", "Connection aborted", "Connection refused", "Not connected", "Already connected", "Connection closed", "Initialization error (interapplication manager)", "Bad occurrence", "Wait on unbound occurrence handler", "Occurrence queue overflow", "Datalog type conflict", "Unused", "Unrecognized type (interapplication manager)", "Memory corrupt", "Failed to make temporary DLL", "Old CIN version", "Drag socket not found", "Failed to load drop-object", "Failed to register OLE object", "Failed to release OLE object", "Format specifier type mismatch", "Unknown format specifier", "Too few format specifiers", "Too many format specifiers", "Scan failed", "Newer CIN version", "Error converting to variant", "Runtime menu error", "Password tampered", "Variant attribute not found", "Incompatible variant data type", "Event data is not available", "Event Store is not present", "Occurrence is not found", "Event Queue is not created", "Event info is not available", "Refnum passed is NULL", "Error retrieving Class GUID", "Error retrieving CoClass GUID", "Error retrieving TypeLib GUID.", "Bad built application magic bytes.", "Specific driver is different from the specific driver associated with the Logical Name.", "There is no session opened to the class driver.", "Max Error", "MAX - Error with config objects", "MAX - Error loading configuration", "MAX - Group not supported"]
        # "Current State"
        # "Handle mistyped state name (developer tool)"
        n112 = Format Into String(format string="Software Exception: Unhandled State \"%s\"." ("message"), error in=w358, w353) -> (resulting string=w361:string, error out=w360:errorcluster)  [unwired: 1 in]
        n113 = call <vilib>:"Error Cluster From Error Code.vi"("show call chain? (False)"=TRUE, "error in (no error)"=w360, "error message (\"\")"=w361, "error code (0)"=w362) -> ("error out"=w359:errorcluster)  [unwired: 5 in]
        n114 = call <vilib>:"Add State(s) to Queue__JKI_lib_State_Machine.vi"("State(s) in (\"\")"=w357) -> ("States Out"=w356:string)  [unwired: 14 in]
      }
      frame "Error Handler" {
        # "Unhandled Error -- Display it"
        # "Clear error"
        n115 = call <vilib>:"General Error Handler.vi"("error in (no error)"=w366) -> ()  [unwired: 10 in, 5 out]
        n116 = call <vilib>:"Add State(s) to Queue__JKI_lib_State_Machine.vi"("State(s) in Front (\"\")"="/* Post Error States", "State(s) in (\"\")"=w370) -> ("States Out"=w369:string)  [unwired: 13 in]
      }
      frame "Exit" {
      }
      frame "---------- Data ----------" {
        n117 = call <vilib>:"Add State(s) to Queue__JKI_lib_State_Machine.vi"("State(s) in (\"\")"=w380) -> ("States Out"=w379:string)  [unwired: 14 in]
      }
      frame "Data: Initialize" {
        w384 = path ""  # log file path
        w387 = string[] []  # Headers in Logfile
        n118 = property class="MainApplication.lvclass"(reference=w390) -> ("Dynamic CVT"=w389:T35, "MasterConfiguration*"=w386:T5)  [unwired: 1 in, 2 out]
        n119 = Unbundle By Name(w386) -> ("EventLoggerConfiguration.LogFolderPath"=w382:path)
        n120 = Bundle("log file path"=w384, "Dynamic CVT"=w389, "LogFolderPath"=w382, "Headers in Logfile"=w387) -> (w385:T36)  [unwired: 1 in]
      }
      frame "---------- Events ----------" {
      }
      frame "Events: Register Events" {
        n121 = register-events(w395) -> (reference out=w396:refnum<event-registration>)  [unwired: 2 in, 1 out]
        n122 = call <vilib>:"Add State(s) to Queue__JKI_lib_State_Machine.vi"("State(s) in (\"\")"=w400) -> ("States Out"=w399:string)  [unwired: 14 in]
      }
      frame "------ Action--------" {
        n123 = call <vilib>:"Add State(s) to Queue__JKI_lib_State_Machine.vi"("State(s) in (\"\")"=w405) -> ("States Out"=w404:string)  [unwired: 14 in]
      }
      frame "Log: Log Status" {
        n124 = Unbundle By Name(w407) -> ("log file path"=w409:path, "Headers in Logfile"=w413:string[], "Dynamic CVT"=w414:T35)
        n125 = call "Log Status Values in file.vi"("error in (no error)"=w412, "Dynamic CVT"=w414, "Headers in Logfile"=w413, "Log File Path"=w409) -> ("error out"=w411:errorcluster, "New Headers"=w408:string[])  [unwired: 5 in, 1 out]
        n126 = Bundle By Name(cluster=w407, "Headers in Logfile"=w408) -> (w406:T36)
      }
      frame "Log: Check File Size" {
        # "If File size is greater than 5MB, Move the event log to Archive and  use a new file for further logging"
        n127 = Unbundle By Name(w417) -> ("LogFolderPath"=w423:path, "log file path"=w425:path)
        n128 = Get File Size(file=w425, error in=w430) -> (size (in bytes)=w429:i64, 0:w422:errorcluster)  [unwired: 1 out]
        n129 = Divide(x=w429, y=i64 1000000) -> (x/y=w427:dbl)
        n130 = Greater Or Equal?(x=w427, y=5.0) -> (x >= y?=w424:bool)
        n131 = case shown="False" w424 {
          tunnel: w425 -> [_ w445]
          tunnel: w423 -> [_ w444]
          tunnel: w422 -> [w433 w440]
          tunnel: [w433 w438] -> w421
          tunnel: [_ "Log: Generate File name"] -> w418
          tunnel: w417 -> [w432 w436]
          tunnel: [w432 w435] -> w416
          frame False {
          }
          frame True {
            n132 = Build Path(base path=w444, name or relative path="Archive") -> (appended path=w442:path)
            n133 = Bundle By Name(cluster=w436, "Headers in Logfile"=string[] []) -> (w435:T36)
            n134 = call <userlib>:"Create Dir if Non-Existant__ogtk.vi"("error in (no error)"=w440, "Directory Path"=w442) -> ("error out"=w439:errorcluster, "dup Directory Path"=w441:path)  [unwired: 7 in, 1 out]
            n135 = Move(source path=w445, error in=w439, 10:w441) -> (error out=w438:errorcluster)  [unwired: 2 in, 2 out]
          }
        }
        n136 = call <vilib>:"Add State(s) to Queue__JKI_lib_State_Machine.vi"("State(s) in Front (\"\")"=w418, "State(s) in (\"\")"=w420) -> ("States Out"=w419:string)  [unwired: 13 in]
      }
      frame "Log: Generate File name" {
        n137 = Unbundle By Name(w447) -> ("LogFolderPath"=w453:path)
        n138 = Get Date/Time In Seconds() -> (seconds since 1Jan1904=w454:timestamp)
        n139 = Format Into String(format string="%s\\\\EventLog_%<%m%Y%d_%H%M%S>T.csv", error in=w452, w453, w454) -> (resulting string=w449:string, error out=w451:errorcluster)  [unwired: 1 in]
        n140 = String To Path(string=w449) -> (path=w448:path)
        n141 = Bundle By Name(cluster=w447, "log file path"=w448) -> (w446:T36)
      }
    }
  }
  n142 = Merge Errors(w3, w2) -> (w1:errorcluster)
  n143 = call "NotifyStop.vi"("error in (no error)"=w1, "index"=9) -> ("error out"=→"error out":errorcluster)  [unwired: 9 in]
  "Event Logger out" <- "Event Logger in"
